vi "Read Execution time.vi"(11 "Method Result In":refnum<class "Method Result.lvclass">) -> (1 "Execution time string":string, 2 "Execution time":dbl, 3 "Method Result Out":refnum<class "Method Result.lvclass">)   [LabVIEW 2020, in "Method Result.lvclass"]
uses:
  Method Result.lvclass
  Method Result.lvclass/Method Result.ctl
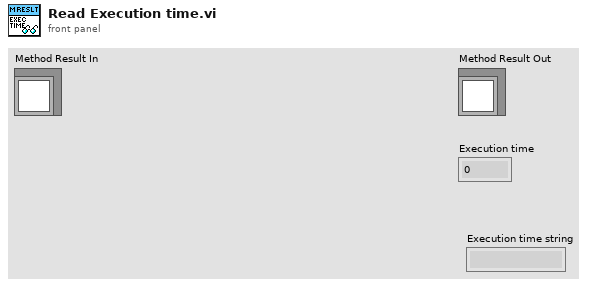
[diagram p1: front panel]
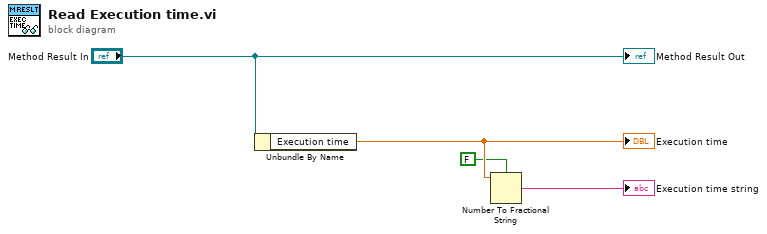
[diagram p0: block diagram]
diagram:
  n1 = Unbundle By Name("Method Result In") -> ("Execution time"=w3:dbl)
  "Execution time" <- w3
  n2 = Number To Fractional String(use system decimal point (T)=FALSE, number=w3) -> (F-format string=→"Execution time string":string)  [unwired: 2 in]
  "Method Result Out" <- "Method Result In"
